vi "write_to_output.vi"(10 "setpoint":dbl, 11 ".NET Refnum in":refnum<k24>) -> (3 ".NET Refnum out":refnum<k24>)   [LabVIEW 2015]
uses:
  C:/Program Files/National Instruments/LabVIEW 2015/vi.lib/ULx/ULx_LV.dll
  <vilib>/ULx/Write.llb/ULx Write (Analog 1D DBL 1Chan 1Samp).vi
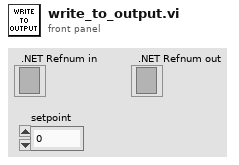
[diagram p1: front panel]
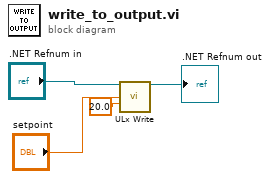
[diagram p0: block diagram]
diagram:
  n1 = call-poly <vilib>:"ULx Write.vi"("task in"=".NET Refnum in", "data"="setpoint", "timeout"=20.0) -> ("task out"=→".NET Refnum out":refnum<k24>)  [unwired: 10 in, 2 out]
